vi "Fetch Waveform.vi"(8 "error in (no error)":errorcluster, 11 "Agilent DSO1000 in":refnum<class "Agilent DSO1000.lvclass">) -> (0 "error out":errorcluster, 2 "Waveform Data":waveform(dbl)[](graph), 3 "Agilent DSO1000 out":refnum<class "Agilent DSO1000.lvclass">)   [LabVIEW 2020, in "Agilent DSO1000.lvclass"]
uses:
  Agilent DSO1000.lvclass
  C:/Sandbox/RF Bench/Source Code/WiSpry Test Framework/Instruments/Instrument.lvclass
  Instrument.lvclass/Instrument.ctl
  Instrument.lvclass
  <instrlib>/Agilent DSO1000 Series/Agilent DSO1000 Series.lvlib
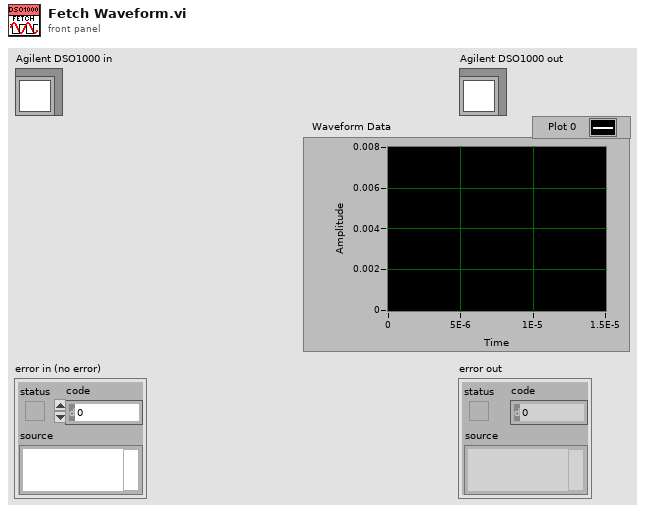
[diagram p1: front panel]
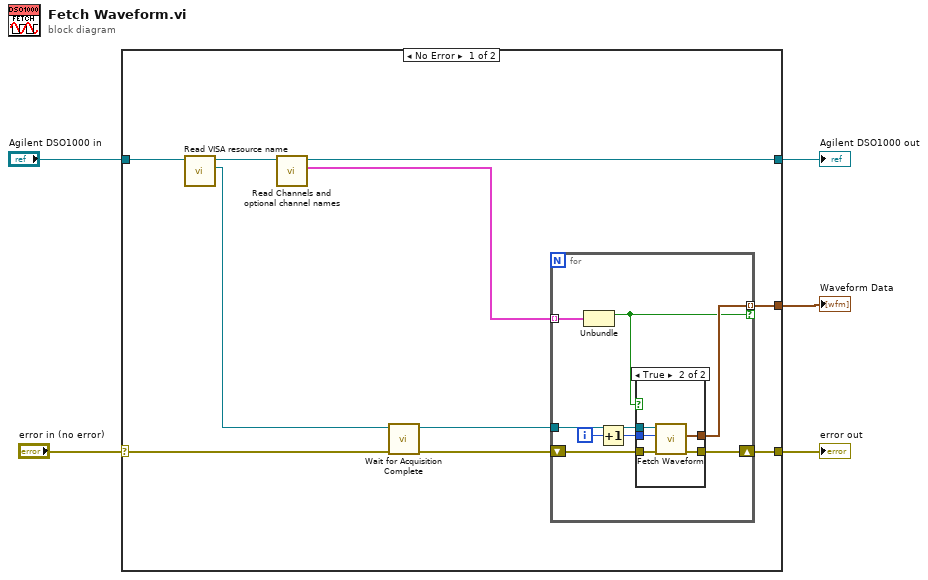
[diagram p0: block diagram]
diagram:
  n1 = case shown="No Error" "error in (no error)" {
    selector: "error in (no error)" -> [w9 w31]
    tunnel: [w10 w31] -> w5
    tunnel: [w13 w30] -> w4
    tunnel: "Agilent DSO1000 in" -> [w15 w30]
    tunnel: [w11 _] -> w3
    frame No Error {
      n2 = call "Read VISA resource name.vi"("Instrument in"=w15) -> ("VISA resource name"=w6:refnum<visa-resource-name>, "Instrument out"=w14:refnum<class "Agilent DSO1000.lvclass">)  [unwired: 9 in]
      n3 = call-dynamic "Read Channels and optional channel names.vi"("Oscilloscope in"=w14) -> ("Channels and optional channel names"=w12:cluster{"Enabled":bool, "Channel name":string}[], "Oscilloscope out"=w13:refnum<class "Agilent DSO1000.lvclass">)  [unwired: 9 in]
      n4 = call <instrlib>:"Wait for Acquisition Complete.vi"("error in (no error)"=w9, "VISA resource name"=w6) -> ("error out"=w7:errorcluster, "VISA resource name out"=w8:refnum<visa-resource-name>)  [unwired: 8 in]
      n5 = for {
        tunnel: w12 -> [w23] mode=indexing
        shift-right: [w19] -> w10
        shift-left: w7 -> [w21]
        tunnel: w8 -> [w20]
        tunnel: [w18] -> w11 mode=indexing if=w16
        i -> [w22]
        n6 = Unbundle(w23) -> ("Enabled"=w16:bool)  [unwired: 1 out]
        n7 = Increment(x=w22) -> (x+1=w17:i32)
        n8 = case shown="True" w16 {
          tunnel: w21 -> [w24 w29]
          tunnel: w20 -> [_ w28]
          tunnel: [w24 w27] -> w19
          tunnel: [_ w26] -> w18
          tunnel: w17 -> [_ w25]
          frame False {
          }
          frame True {
            n9 = call <instrlib>:"Fetch Waveform.vi"("error in (no error)"=w29, "Channel (1: Channel 1)"=w25, "VISA resource name"=w28) -> ("error out"=w27:errorcluster, "Waveform Data"=w26:waveform(dbl))  [unwired: 6 in, 1 out]
          }
        }
      }
    }
    frame Error {
    }
  }
  "error out" <- w5
  "Agilent DSO1000 out" <- w4
  "Waveform Data" <- w3
